vi "SerialMove setpointXY_ASI.vi"(2 "VISA resource name":refnum<visa-resource-name>="COM7", 3 "error in":errorcluster, 4 "Y":dbl, 5 "X":dbl) -> (0 "error out":errorcluster)   [LabVIEW 2015]
uses:
  <vilib>/Instr/_visa.llb/VISA Flush IO Buffer Mask.ctl
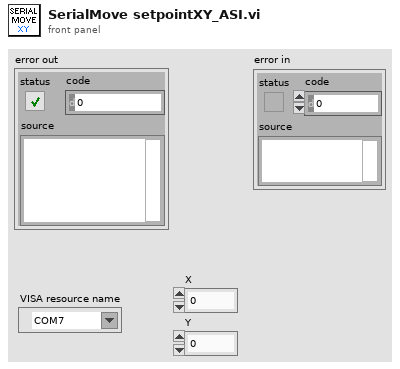
[diagram p1: front panel]
types:
  T1 = typedef "VISA Flush IO Buffer Mask.ctl" = u16
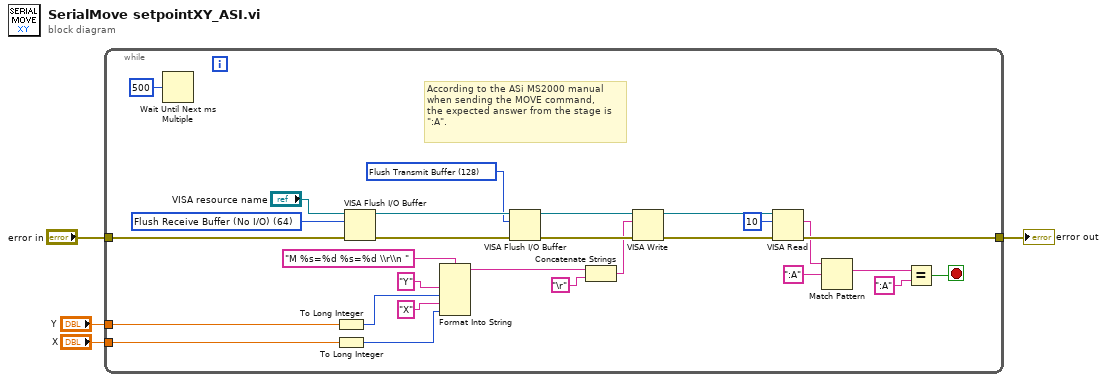
[diagram p0: block diagram]
diagram:
  n1 = while {
    tunnel: "Y" -> [w11]
    tunnel: "X" -> [w10]
    tunnel: "error in" -> [w23]
    tunnel: [w15] -> w4
    stop <- w5 stop-if-true
    w26 = T1 128 items=["Flush Receive Buffer"=16, "Write Transmit Buffer to Device"=32, "Flush Receive Buffer (No I/O)"=64, "Flush Transmit Buffer"=128] ("Mask")
    w29 = T1 64 items=["Flush Receive Buffer"=16, "Write Transmit Buffer to Device"=32, "Flush Receive Buffer (No I/O)"=64, "Flush Transmit Buffer"=128] ("Mask")
    # "According to the ASi MS2000 manual\nwhen sending the MOVE command, \nthe expected answer from the stage is\n\":A\"."
    n2 = Wait Until Next ms Multiple(millisecond multiple=u32 500) -> ()  [unwired: 1 out]
    n3 = To Long Integer(number=w11) -> (32bit integer=w12:i32)
    n4 = To Long Integer(number=w10) -> (32bit integer=w13:i32)
    n5 = VISA Flush I/O Buffer(VISA resource name="VISA resource name", mask (16)=w29, error in (no error)=w23) -> (VISA resource name out=w27:refnum<visa-resource-name>, error out=w28:errorcluster)
    n6 = Format Into String "Format Into String"(format string="M %s=%d %s=%d \\r\\n ", "Y" ("Axis"), w12, "X" ("Axis"), w13) -> (resulting string=w21:string)  [unwired: 2 in, 1 out]
    n7 = VISA Flush I/O Buffer(VISA resource name=w27, mask (16)=w26, error in (no error)=w28) -> (VISA resource name out=w24:refnum<visa-resource-name>, error out=w25:errorcluster)
    n8 = Concatenate Strings(w21, "\r") -> (w19:string)
    n9 = VISA Write(VISA resource name=w24, write buffer=w19, error in (no error)=w25) -> (VISA resource name out=w32:refnum<visa-resource-name>, error out=w22:errorcluster)  [unwired: 1 out]
    n10 = VISA Read(VISA resource name=w32, byte count=u32 10, error in (no error)=w22) -> (read buffer=w8:string, error out=w15:errorcluster)  [unwired: 2 out]
    n11 = Match Pattern(string=w8, regular expression=":A" ("y")) -> (match substring=w7:string)  [unwired: 1 in, 3 out]
    n12 = Equal?(x=w7, y=":A") -> (x = y?=w5:bool)
  }
  "error out" <- w4
